vi "SimpleDialog.vi"() -> (19 "error out":errorcluster)   [LabVIEW 2018, in "LcWebView.lvclass"]
uses:
  LcWebView.lvclass
  <vilib>/event_ctls.llb/eventvkey.ctl
  C:/Projects/LcWebView2/LcWebView/LcWebView_class/data/Microsoft.Web.WebView2.WinForms.dll
  data/Microsoft.Web.WebView2.WinForms.dll
panel:
  in  "Webview container":refnum<k24>(container)
  out "String":string
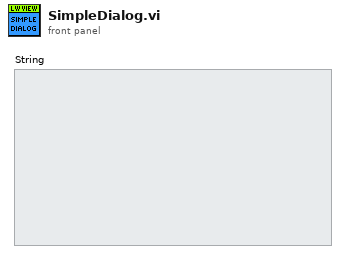
[diagram p1: front panel]
types:
  T1 = cluster{"title":string, "showDenyButton":bool, "showCancelButton":bool, "confirmButtonText":string, "denyButtonText":string}
  T2 = typedef "eventvkey.ctl" = enum16{"ASCII", "Enter", "Return", "Shift", "Ctrl", "Alt", "Cmd", "Opt", "Caps", "NumLock", "Clear", "Break", "Up", "Down", "Left", "Right", "Insert", "Delete", "Home", "End", "PageUp", "PageDown", "Escape", "Help", "Pause", "ScrollLock", "F1", "F2", "F3", "F4", "F5", "F6", "F7", "F8", "F9", "F10", "F11", "F12", "F13", "F14", "F15", "F16", "F17", "F18", "F19", "F20", "F21", "F22", "F23", "F24", "Play", "VolumeUp", "VolumeDown", "Mute", "Two Byte Char"}
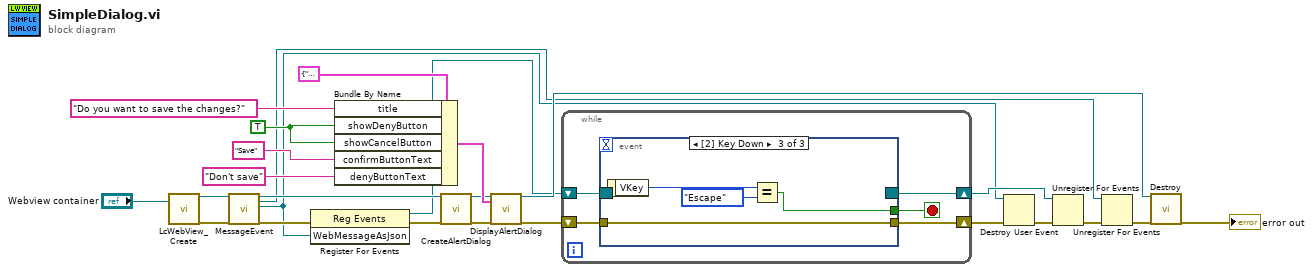
[diagram p0: block diagram]
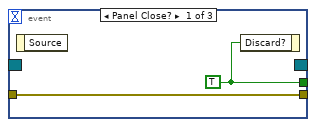
[diagram p2: hidden frame]
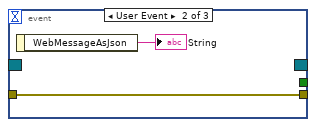
[diagram p3: hidden frame]
diagram:
  w22 = TRUE ("showDenyButton")
  n1 = call "LcWebView_Create.vi"("Webview container"="Webview container") -> ("reference out"=w12:refnum<class "LcWebView.lvclass">, "Error Out"=w11:errorcluster)  [unwired: 11 in, 6 out]
  n2 = call "MessageEvent.vi"("reference in"=w12, "error in (no error)"=w11) -> ("reference out"=w13:refnum<class "LcWebView.lvclass">, "Event Callback"=w4:refnum<k27>, "WebMessageAsJson"=w2:refnum<user-event>, "error out"=w10:errorcluster)  [unwired: 14 in]
  n3 = register-events(error in=w10, w2) -> (reference out=w6:refnum<event-registration>, error out=w9:errorcluster)  [unwired: 1 in]
  n4 = Bundle By Name(cluster=T1 {"title"="", "showDenyButton"=FALSE, "showCancelButton"=FALSE, "confirmButtonText"="", "denyButtonText"=""}, "title"="Do you want to save the changes?", "showDenyButton"=w22, "showCancelButton"=w22, "confirmButtonText"="Save", "denyButtonText"="Don't save") -> (w19:T1)
  n5 = call-dynamic "CreateAlertDialog.vi"("reference in"=w13, "Error In"=w9) -> ("reference out"=w14:refnum<class "LcWebView.lvclass">, "Error Out"=w8:errorcluster)  [unwired: 16 in]
  n6 = call-dynamic "DisplayAlertDialog.vi"("reference in"=w14, "Message"=w19, "Error In"=w8) -> ("reference out"=w15:refnum<class "LcWebView.lvclass">, "Error Out"=w7:errorcluster)  [unwired: 14 in, 1 out]
  n7 = while {
    shift-right: [w30] -> w3
    shift-left: w7 -> [w29]
    shift-right: [w27] -> w5
    shift-left: w6 -> [w28]
    stop <- w26 stop-if-true
    n8 = event shown="[2] Key Down" {
      selector: w28 -> [_ _ _]
      dyn-events: [_ _ _] -> w27
      timeout: _ -> [_ _ _]
      tunnel: [w32 _ w36] -> w26
      tunnel: w29 -> [w31 w33 w35]
      tunnel: [w31 w33 w35] -> w30
      event Panel Close? {
        w32 = TRUE ("Discard?")
        n9 = event-data() -> ()  [unwired: 1 in, 1 out]
        n10 = event-data("Discard?"=w32) -> ()  [unwired: 1 in, 1 out]
      }
      event User Event {
        n11 = event-data() -> ("WebMessageAsJson"=→"String":string)  [unwired: 1 in]
      }
      event Key Down {
        n12 = event-data() -> ("VKey"=w38:T2)  [unwired: 1 in]
        n13 = Equal?(x=w38, y=eventvkey."Escape") -> (x = y?=w36:bool)
      }
    }
  }
  n14 = Destroy User Event(user event=w2, error in=w3) -> (error out=w16:errorcluster)
  n15 = Unregister For Events(event registration refnum=w5, error in=w16) -> (error out=w18:errorcluster)
  n16 = Unregister For Events(event registration refnum=w4, error in=w18) -> (error out=w17:errorcluster)
  n17 = call-dynamic "Destroy.vi"("reference in"=w15, "Error In"=w17) -> ("Error Out"=→"error out":errorcluster)  [unwired: 16 in, 1 out]
